vi "LoadOrCreateATeststepIniCfg.vi"(8 "error in":errorcluster, 10 "Tree Refnum":refnum<vi>, 11 "Tbl Refnum in":refnum<vi>) -> (0 "error out":errorcluster, 1 "cfg file refnum out":refnum<file>, 2 "Tree Refnum out":refnum<vi>, 3 "Tbl Refnum out":refnum<vi>)   [LabVIEW 2010]
uses:
  <vilib>/Utility/miscctls.llb/LVRowAndColumnTypeDef.ctl
panel:
  out "All Tags":string[](array[string])
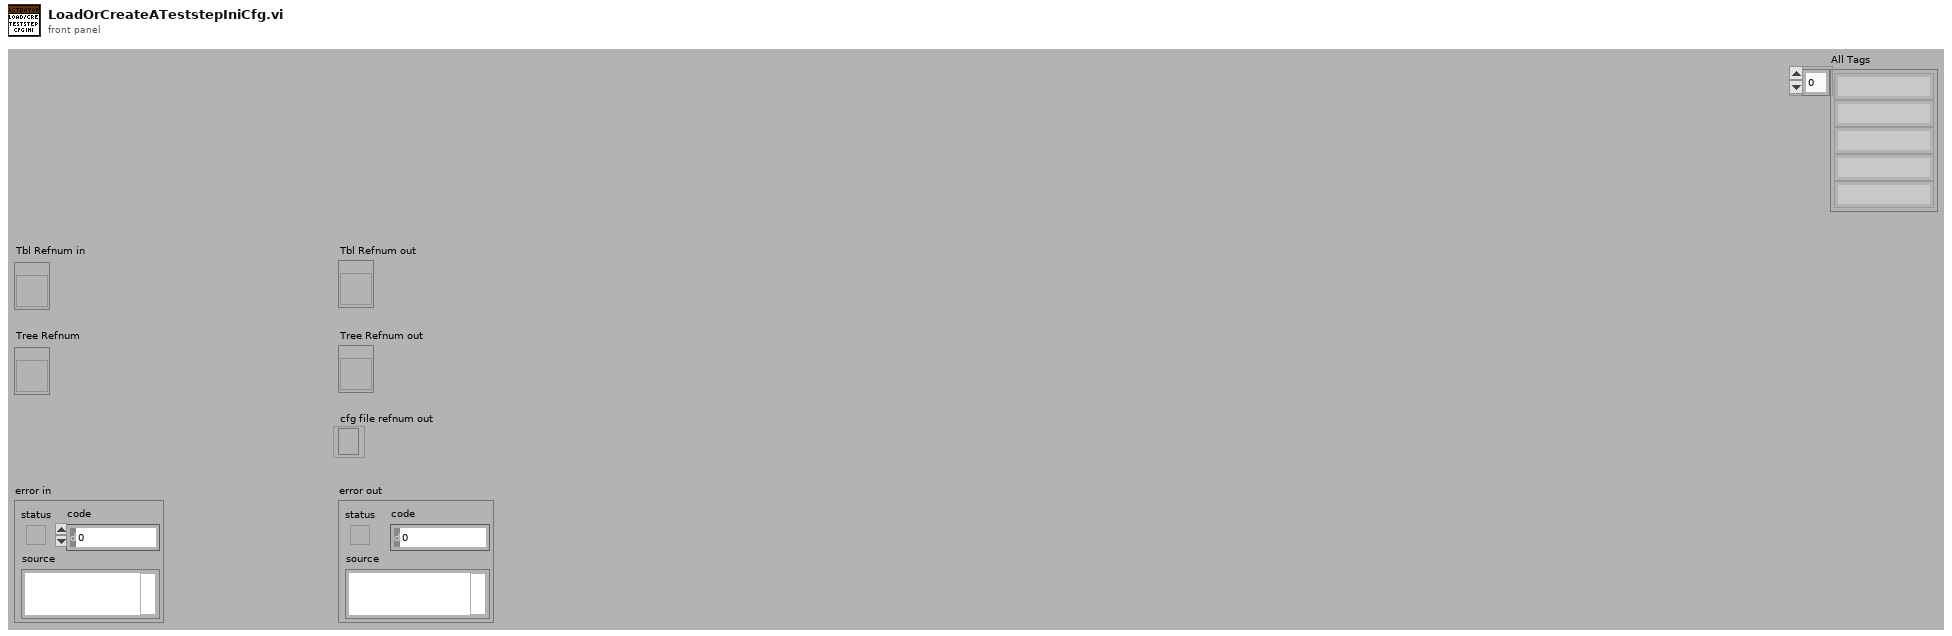
[diagram p1: front panel]
types:
  T1 = typedef "LVRowAndColumnTypeDef.ctl" = cluster{"Row":i32, "Column":i32}
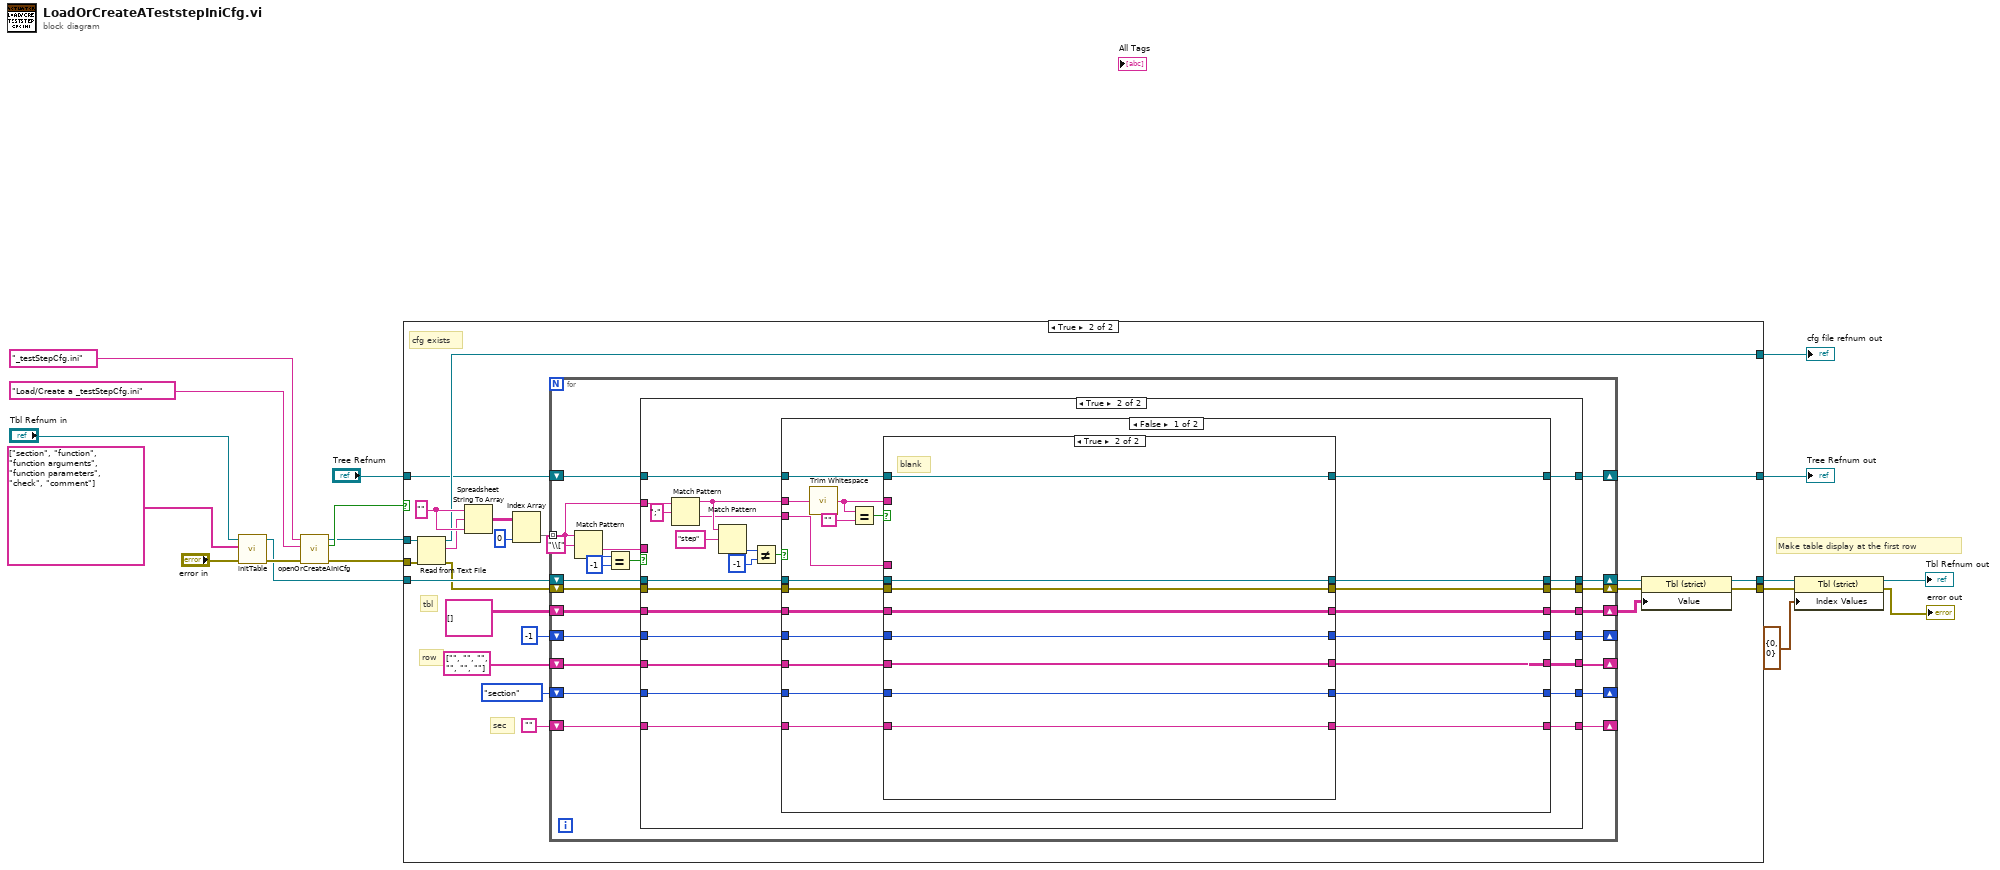
[diagram p0: block diagram]
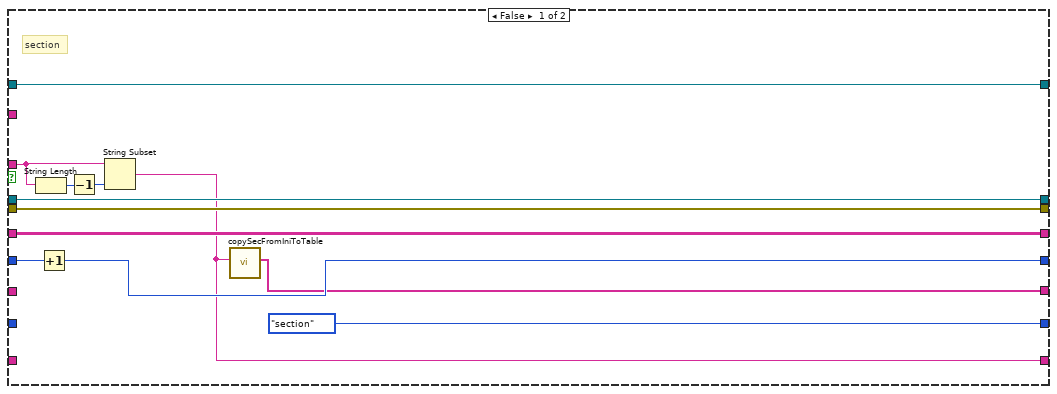
[diagram p3: hidden frame]
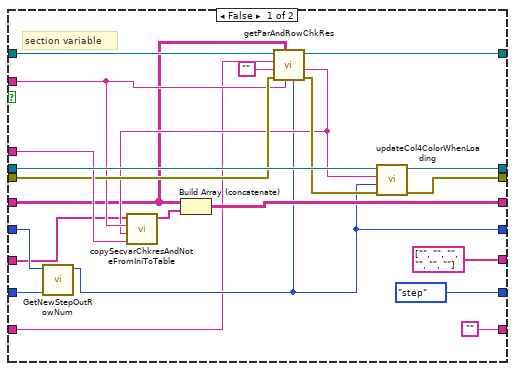
[diagram p4: hidden frame]
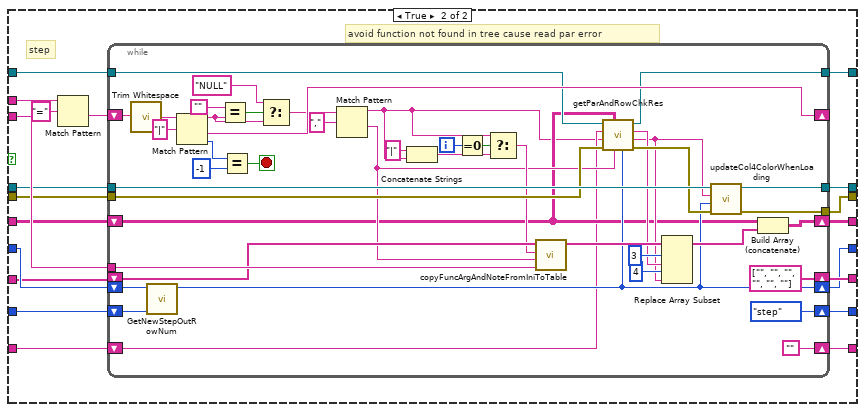
[diagram p5: hidden frame]
diagram:
  # "Make table display at the first row"
  n1 = call "initTable.vi"("error in"="error in", "Column Header Strings[]"=string[] ["section", "function", "function arguments", "function parameters", "check", "comment"] ("Row Header Strings[]"), "Tbl Refnum in"="Tbl Refnum in") -> ("error out"=w13:errorcluster, "Tbl Refnum out"=w9:refnum<vi>)  [unwired: 7 in]
  n2 = call "openOrCreateAIniCfg.vi"("error in"=w13, "prompt"="Load/Create a _testStepCfg.ini", "default name"="_testStepCfg.ini") -> ("error out"=w10:errorcluster, "exists"=w12:bool, "ini refnum out"=w11:refnum<file>)  [unwired: 6 in]
  n3 = case shown="True" w12 {
    tunnel: w11 -> [w22 w40]
    tunnel: w10 -> [w21 w39]
    tunnel: w9 -> [w20 w37]
    tunnel: [w22 w34] -> w18
    tunnel: [w21 w24] -> w4
    tunnel: [w20 w25] -> w5
    tunnel: "Tree Refnum" -> [w19 w32]
    tunnel: [w19 w31] -> w16
    frame False {
      # "create a new cfg"
    }
    frame True {
      w42 = ""
      # "sec"
      # "row"
      # "tbl"
      # "cfg exists"
      n4 = Read from Text File(file (use dialog)=w40, error in=w39) -> (refnum out=w34:refnum<file>, text=w41:string, error out=w33:errorcluster)  [unwired: 2 in, 1 out]
      n5 = Spreadsheet String To Array(format string=w42, spreadsheet string=w41, array type (2D Dbl)=w42) -> (array=w43:string[][])  [unwired: 1 in]
      n6 = Index Array(array=w43, index (col)=0 ("disabled index (col)")) -> (element=w38:string[])  [unwired: 1 in]
      n7 = for {
        tunnel: w38 -> [w60] mode=indexing
        shift-right: [w58] -> _
        shift-left: -1 -> [w62]
        shift-right: [w57] -> _
        shift-left: enum16{"section", "step"}."section" -> [w56]
        shift-right: [w55] -> w27
        shift-left: w33 -> [w54]
        shift-right: [w53] -> w28
        shift-left: w37 -> [w59]
        shift-right: [w51] -> w31
        shift-left: w32 -> [w52]
        shift-right: [w49] -> w26
        shift-left: string[][] [] -> [w50]
        shift-right: [w48] -> _
        shift-left: string[] ["", "", "", "", "", ""] -> [w47]
        shift-right: [w46] -> _
        shift-left: "" -> [w45]
        n8 = Match Pattern(string=w60, regular expression="\\[") -> (after substring=w61:string, offset past match=w65:i32)  [unwired: 1 in, 2 out]
        n9 = Equal?(x=w65, y=-1) -> (x = y?=w63:bool)
        n10 = case shown="True" w63 {
          tunnel: w62 -> [w75 w97]
          tunnel: [w70 w96] -> w58
          tunnel: w61 -> [w78 _]
          tunnel: w60 -> [_ w90]
          tunnel: w59 -> [w71 w98]
          tunnel: [enum16{"section", "step"}."section" w95] -> w57
          tunnel: w56 -> [_ w94]
          tunnel: w54 -> [w72 w93]
          tunnel: [w72 w92] -> w55
          tunnel: [w71 w91] -> w53
          tunnel: w52 -> [w73 w87]
          tunnel: [w73 w86] -> w51
          tunnel: w50 -> [w68 w84]
          tunnel: [w68 w83] -> w49
          tunnel: [w69 w81] -> w48
          tunnel: w47 -> [_ w82]
          tunnel: [w67 w79] -> w46
          tunnel: w45 -> [_ w80]
          frame False {
            # "section"
            n11 = String Length(string=w78) -> (length=w77:i32)
            n12 = Increment(x=w75) -> (x+1=w70:i32)
            n13 = Decrement(x=w77) -> (x-1=w76:i32)
            n14 = String Subset(string=w78, length (rest)=w76) -> (substring=w67:string)  [unwired: 1 in]
            n15 = call "copySecFromIniToTable.vi"("valInCol0"=w67) -> ("arrWithSec"=w69:string[])  [unwired: 10 in]
          }
          frame True {
            n16 = Match Pattern(string=w90, regular expression=";") -> (before substring=w88:string, after substring=w85:string)  [unwired: 1 in, 2 out]
            n17 = Match Pattern(string=w88, regular expression="step") -> (offset past match=w100:i32)  [unwired: 1 in, 3 out]
            n18 = Not Equal?(x=w100, y=-1) -> (x != y?=w102:bool)
            n19 = case shown="False" w102 {
              tunnel: w88 -> [w123 w172]
              tunnel: w98 -> [w121 w165]
              tunnel: w97 -> [w119 w170]
              tunnel: [w114 w158] -> w96
              tunnel: [w113 w157] -> w95
              tunnel: w94 -> [w118 w169]
              tunnel: w93 -> [w120 w166]
              tunnel: [w116 w164] -> w92
              tunnel: [w115 w163] -> w91
              tunnel: w87 -> [w112 w167]
              tunnel: [w111 w155] -> w86
              tunnel: w85 -> [w117 w168]
              tunnel: w84 -> [w108 w162]
              tunnel: [w107 w160] -> w83
              tunnel: w82 -> [w106 w159]
              tunnel: [w105 w161] -> w81
              tunnel: w80 -> [w104 w156]
              tunnel: [w103 w154] -> w79
              frame False {
                n20 = call <vilib>:"Trim Whitespace.vi"("string"=w123) -> ("trimmed string"=w109:string)  [unwired: 1 in]
                n21 = Equal?(x=w109, y="") -> (x = y?=w122:bool)
                n22 = case shown="True" w122 {
                  tunnel: w121 -> [w140 w153]
                  tunnel: w120 -> [w134 w152]
                  tunnel: w119 -> [w145 w151]
                  tunnel: w118 -> [w144 w150]
                  tunnel: w117 -> [w139 _]
                  tunnel: [w141 w152] -> w116
                  tunnel: [w142 w153] -> w115
                  tunnel: [w128 w151] -> w114
                  tunnel: [enum16{"section", "step"}."step" w150] -> w113
                  tunnel: [w135 w149] -> w111
                  tunnel: w112 -> [w136 w149]
                  tunnel: w109 -> [w132 _]
                  tunnel: w108 -> [w127 w148]
                  tunnel: [w138 w148] -> w107
                  tunnel: w106 -> [w129 w147]
                  tunnel: [string[] ["", "", "", "", "", ""] w147] -> w105
                  tunnel: ["" w146] -> w103
                  tunnel: w104 -> [w126 w146]
                  frame False {
                    # "section variable"
                    n23 = call "GetNewStepOutRowNum.vi"("lastStat"=w144, "lastRowNum"=w145) -> ("outRowNum"=w128:i32)  [unwired: 9 in]
                    n24 = call "getParAndRowChkRes.vi"("Row number"=w128, "arg"=w132, "table"=w127, "error in"=w134, "function"="", "section"=w126, "Tree Refnum in"=w136) -> ("error out"=w133:errorcluster, "Check result"=w131:string, "Tree Refnum out"=w135:refnum<vi>)  [unwired: 1 in, 1 out]
                    n25 = call "copySecvarChkresAndNoteFromIniToTable.vi"("valInCol5"=w139, "valInCol4"=w131, "valInCol2"=w132, "arrayAtSameRow"=w129) -> ("arrWithSecvar&Chkres&Note"=w130:string[])  [unwired: 7 in]
                    n26 = Build Array (concatenate)(w127, w130) -> (w138:string[][])
                    n27 = call "updateCol4ColorWhenLoading.vi"("error in"=w133, "rowNum"=w128, "judgeRes"=w131, "Tbl Refnum in"=w140) -> ("error out"=w141:errorcluster, "Tbl Refnum Out"=w142:refnum<vi>)  [unwired: 6 in]
                  }
                  frame True {
                    # "blank"
                  }
                }
              }
              frame True {
                # "avoid function not found in tree cause read par error"
                # "step"
                n28 = Match Pattern(string=w172, regular expression="=") -> (after substring=w171:string)  [unwired: 1 in, 3 out]
                n29 = while {
                  tunnel: w168 -> [w214]
                  tunnel: w167 -> [w186]
                  tunnel: w166 -> [w185]
                  tunnel: w165 -> [w211]
                  tunnel: [w210] -> w164
                  tunnel: [w209] -> w163
                  shift-right: [w198] -> _
                  shift-left: w171 -> [w203]
                  shift-right: [w199] -> w160
                  shift-left: w162 -> [w177]
                  shift-right: [string[] ["", "", "", "", "", ""]] -> w161
                  shift-left: w159 -> [w192]
                  shift-right: [w178] -> w158
                  shift-left: w170 -> [w216]
                  shift-right: [enum16{"section", "step"}."step"] -> w157
                  shift-left: w169 -> [w215]
                  tunnel: [w181] -> w155
                  shift-right: [""] -> w154
                  shift-left: w156 -> [w176]
                  i -> [w196]
                  stop <- w200 stop-if-true
                  n30 = call <vilib>:"Trim Whitespace.vi"("string"=w203) -> ("trimmed string"=w205:string)  [unwired: 1 in]
                  n31 = call "GetNewStepOutRowNum.vi"("lastStat"=w215, "lastRowNum"=w216) -> ("outRowNum"=w178:i32)  [unwired: 9 in]
                  n32 = Match Pattern(string=w205, regular expression="|") -> (before substring=w188:string, after substring=w198:string, offset past match=w202:i32)  [unwired: 1 in, 1 out]
                  n33 = Equal?(x="", y=w188) -> (x = y?=w190:bool)
                  n34 = Equal?(x=w202, y=-1) -> (x = y?=w200:bool)
                  n35 = Select(t="NULL", s=w190, f=w188) -> (s? t:f=w187:string)
                  n36 = Match Pattern(string=w187, regular expression=",") -> (before substring=w175:string, after substring=w183:string)  [unwired: 1 in, 2 out]
                  n37 = Concatenate Strings("|", w175) -> (w193:string)
                  n38 = Equal To 0?(x=w196) -> (x = 0?=w195:bool)
                  n39 = Select(t=w175, s=w195, f=w193) -> (s? t:f=w184:string)
                  n40 = call "copyFuncArgAndNoteFromIniToTable.vi"("valInCol5"=w214, "valInCol2"=w183, "valInCol1"=w184, "arrayAtTheSameRow"=w192) -> ("arrWithFunc&Arg&Note"=w207:string[])  [unwired: 7 in]
                  n41 = call "getParAndRowChkRes.vi"("Row number"=w178, "arg"=w183, "table"=w177, "error in"=w185, "function"=w175, "section"=w176, "Tree Refnum in"=w186) -> ("error out"=w182:errorcluster, "Check result"=w179:string, "par"=w180:string, "Tree Refnum out"=w181:refnum<vi>)  [unwired: 1 in]
                  n42 = Replace Array Subset(array=w207, new element #1=w180, index #1=3 ("index"), new element #2=w179, index #2=4 ("index")) -> (w208:string[])
                  n43 = call "updateCol4ColorWhenLoading.vi"("error in"=w182, "rowNum"=w178, "judgeRes"=w179, "Tbl Refnum in"=w211) -> ("error out"=w210:errorcluster, "Tbl Refnum Out"=w209:refnum<vi>)  [unwired: 6 in]
                  n44 = Build Array (concatenate)(w177, w208) -> (w199:string[][])
                }
              }
            }
          }
        }
      }
      n45 = property class="Tbl (strict)"(reference=w28, error in=w27, "Value"=w26) -> (reference out=w25:refnum<vi>, error out=w24:errorcluster)
    }
  }
  "cfg file refnum out" <- w18
  "Tree Refnum out" <- w16
  n46 = property on="Property Node" class="Tbl (strict)"(reference=w5, error in=w4, "Index Values"=T1 {"Row"=0, "Column"=0} ("Active Cell:Active Cell")) -> (reference out=→"Tbl Refnum out":refnum<vi>, error out=→"error out":errorcluster)
